vi "2013_01_04 Durability8 Main.vi"() -> ()   [LabVIEW 2011]
uses:
  MotorTypeDef.ctl
  <vilib>/DAQmx/write.llb/DAQmx Write (Counter Time 1Chan 1Samp).vi
  <vilib>/DAQmx/read.llb/DAQmx Read (Analog 1D Wfm NChan NSamp).vi
  <vilib>/Utility/TradDaqScaling.llb/Convert Thermistor Reading (waveform).vi
  <vilib>/DAQmx/miscellaneous.llb/DAQmx Fill In Error Info.vi
  <vilib>/measure/madcrms.llb/Averaged DC-RMS for N Chan.vi
  <vilib>/measure/NI_MAPro.lvlib
panel:
  out "error out":errorcluster
  in  "File Path":path=path "Durability/fine.lvm"
  out "Voltages":waveform(dbl)[](graph)
  out "Currents":waveform(dbl)[](graph)
  in  "Motor 8":T1 {"Elapsed Time" format="%<%H:%M:%S>t"; "Efficiency" format="%#_3g%%"; "Supply Voltage (V)" format="%#_3f"; "Power Output (W)" format="%#_3g"; "Power Usage (W)" format="%#_3g"; "Torque (mNm)" format="%#_3g"; "RPM" scale=0.0..40000.0 scale format="%#.6p"}
  in  "Motor 7":T1 {"Elapsed Time" format="%<%H:%M:%S>t"; "Efficiency" format="%#_3g%%"; "Supply Voltage (V)" format="%#_3f"; "Power Output (W)" format="%#_3g"; "Power Usage (W)" format="%#_3g"; "Torque (mNm)" format="%#_3g"; "RPM" scale=0.0..40000.0 scale format="%#.6p"}
  in  "Motor 6":T1 {"Elapsed Time" format="%<%H:%M:%S>t"; "Efficiency" format="%#_3g%%"; "Supply Voltage (V)" format="%#_3f"; "Power Output (W)" format="%#_3g"; "Power Usage (W)" format="%#_3g"; "Torque (mNm)" format="%#_3g"; "RPM" scale=0.0..40000.0 scale format="%#.6p"}
  in  "Motor 5":T1 {"Elapsed Time" format="%<%H:%M:%S>t"; "Efficiency" format="%#_3g%%"; "Supply Voltage (V)" format="%#_3f"; "Power Output (W)" format="%#_3g"; "Power Usage (W)" format="%#_3g"; "Torque (mNm)" format="%#_3g"; "RPM" scale=0.0..40000.0 scale format="%#.6p"}
  in  "Motor 4":T1 {"Elapsed Time" format="%<%H:%M:%S>t"; "Efficiency" format="%#_3g%%"; "Supply Voltage (V)" format="%#_3f"; "Power Output (W)" format="%#_3g"; "Power Usage (W)" format="%#_3g"; "Torque (mNm)" format="%#_3g"; "RPM" scale=0.0..40000.0 scale format="%#.6p"}
  in  "Motor 3":T1 {"Elapsed Time" format="%<%H:%M:%S>t"; "Efficiency" format="%#_3g%%"; "Supply Voltage (V)" format="%#_3f"; "Power Output (W)" format="%#_3g"; "Power Usage (W)" format="%#_3g"; "Torque (mNm)" format="%#_3g"; "RPM" scale=0.0..40000.0 scale format="%#.6p"}
  in  "Motor 2":T1 {"Elapsed Time" format="%<%H:%M:%S>t"; "Efficiency" format="%#_3g%%"; "Supply Voltage (V)" format="%#_3f"; "Power Output (W)" format="%#_3g"; "Power Usage (W)" format="%#_3g"; "Torque (mNm)" format="%#_3g"; "RPM" scale=0.0..40000.0 scale format="%#.6p"}
  in  "Motor 1":T1 {"Elapsed Time" format="%<%H:%M:%S>t"; "Efficiency" format="%#_3g%%"; "Supply Voltage (V)" format="%#_3f"; "Power Output (W)" format="%#_3g"; "Power Usage (W)" format="%#_3g"; "Torque (mNm)" format="%#_3g"; "RPM" scale=0.0..40000.0 scale format="%#.6p"}
  out "Motor Temp":dbl(slide) scale=90.0..110.0
  out "Tank Temp":dbl(slide) scale=90.0..110.0
  out "RMS Voltages":waveform(dbl)[](graph)
  out "RMS Currents":waveform(dbl)[](graph)
  in  "Temp Probe\nOn Motor":dbl=1.0
  out "loop time (ms)":u32
  in  "stop":bool
  in  "Unlock PWM":bool=TRUE
  in  "PWM 2":dbl(slide)=100.0 min=0.0 max=100.0 step=5.0 scale=0.0..100.0
  in  "PWM 1":dbl(slide) min=0.0 max=100.0 step=5.0 scale=0.0..100.0
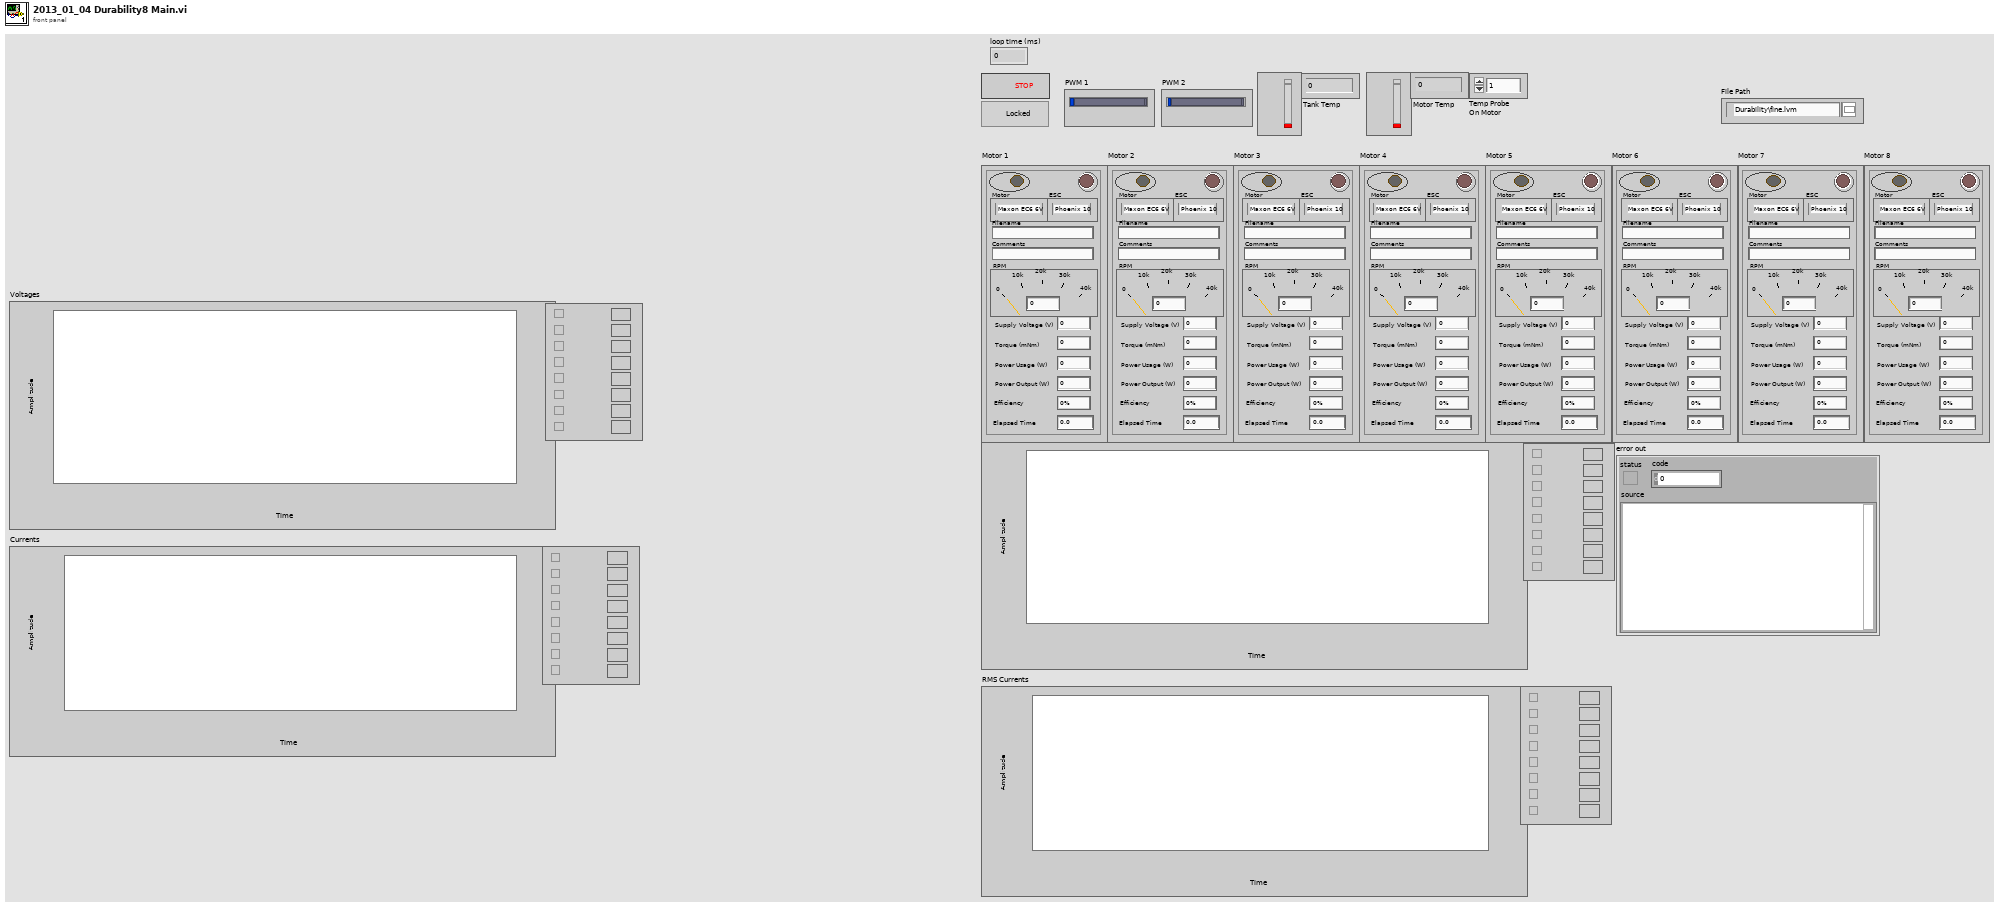
[diagram p1: front panel]
types:
  T1 = typedef "MotorTypeDef.ctl" = cluster{"Enabled":bool, "Fail":bool, "RPM":dbl, "Motor":enum16{"Maxon EC6 6V", "Maxon EC4 6V", "FH 0620 6V", "FH 0620 12V"}, "ESC":enum16{"Phoenix 10", "Maxon", "FH 1801"}, "Torque (mNm)":dbl, "Power Usage (W)":dbl, "Power Output (W)":dbl, "Supply Voltage (V)":dbl, "Efficiency":dbl, "Filename":string, "Comments":string, "Elapsed Time":dbl, "Counter":dbl}
  T2 = enum8{"Enabled", "Disabled", "Disabled and Grayed Out"}
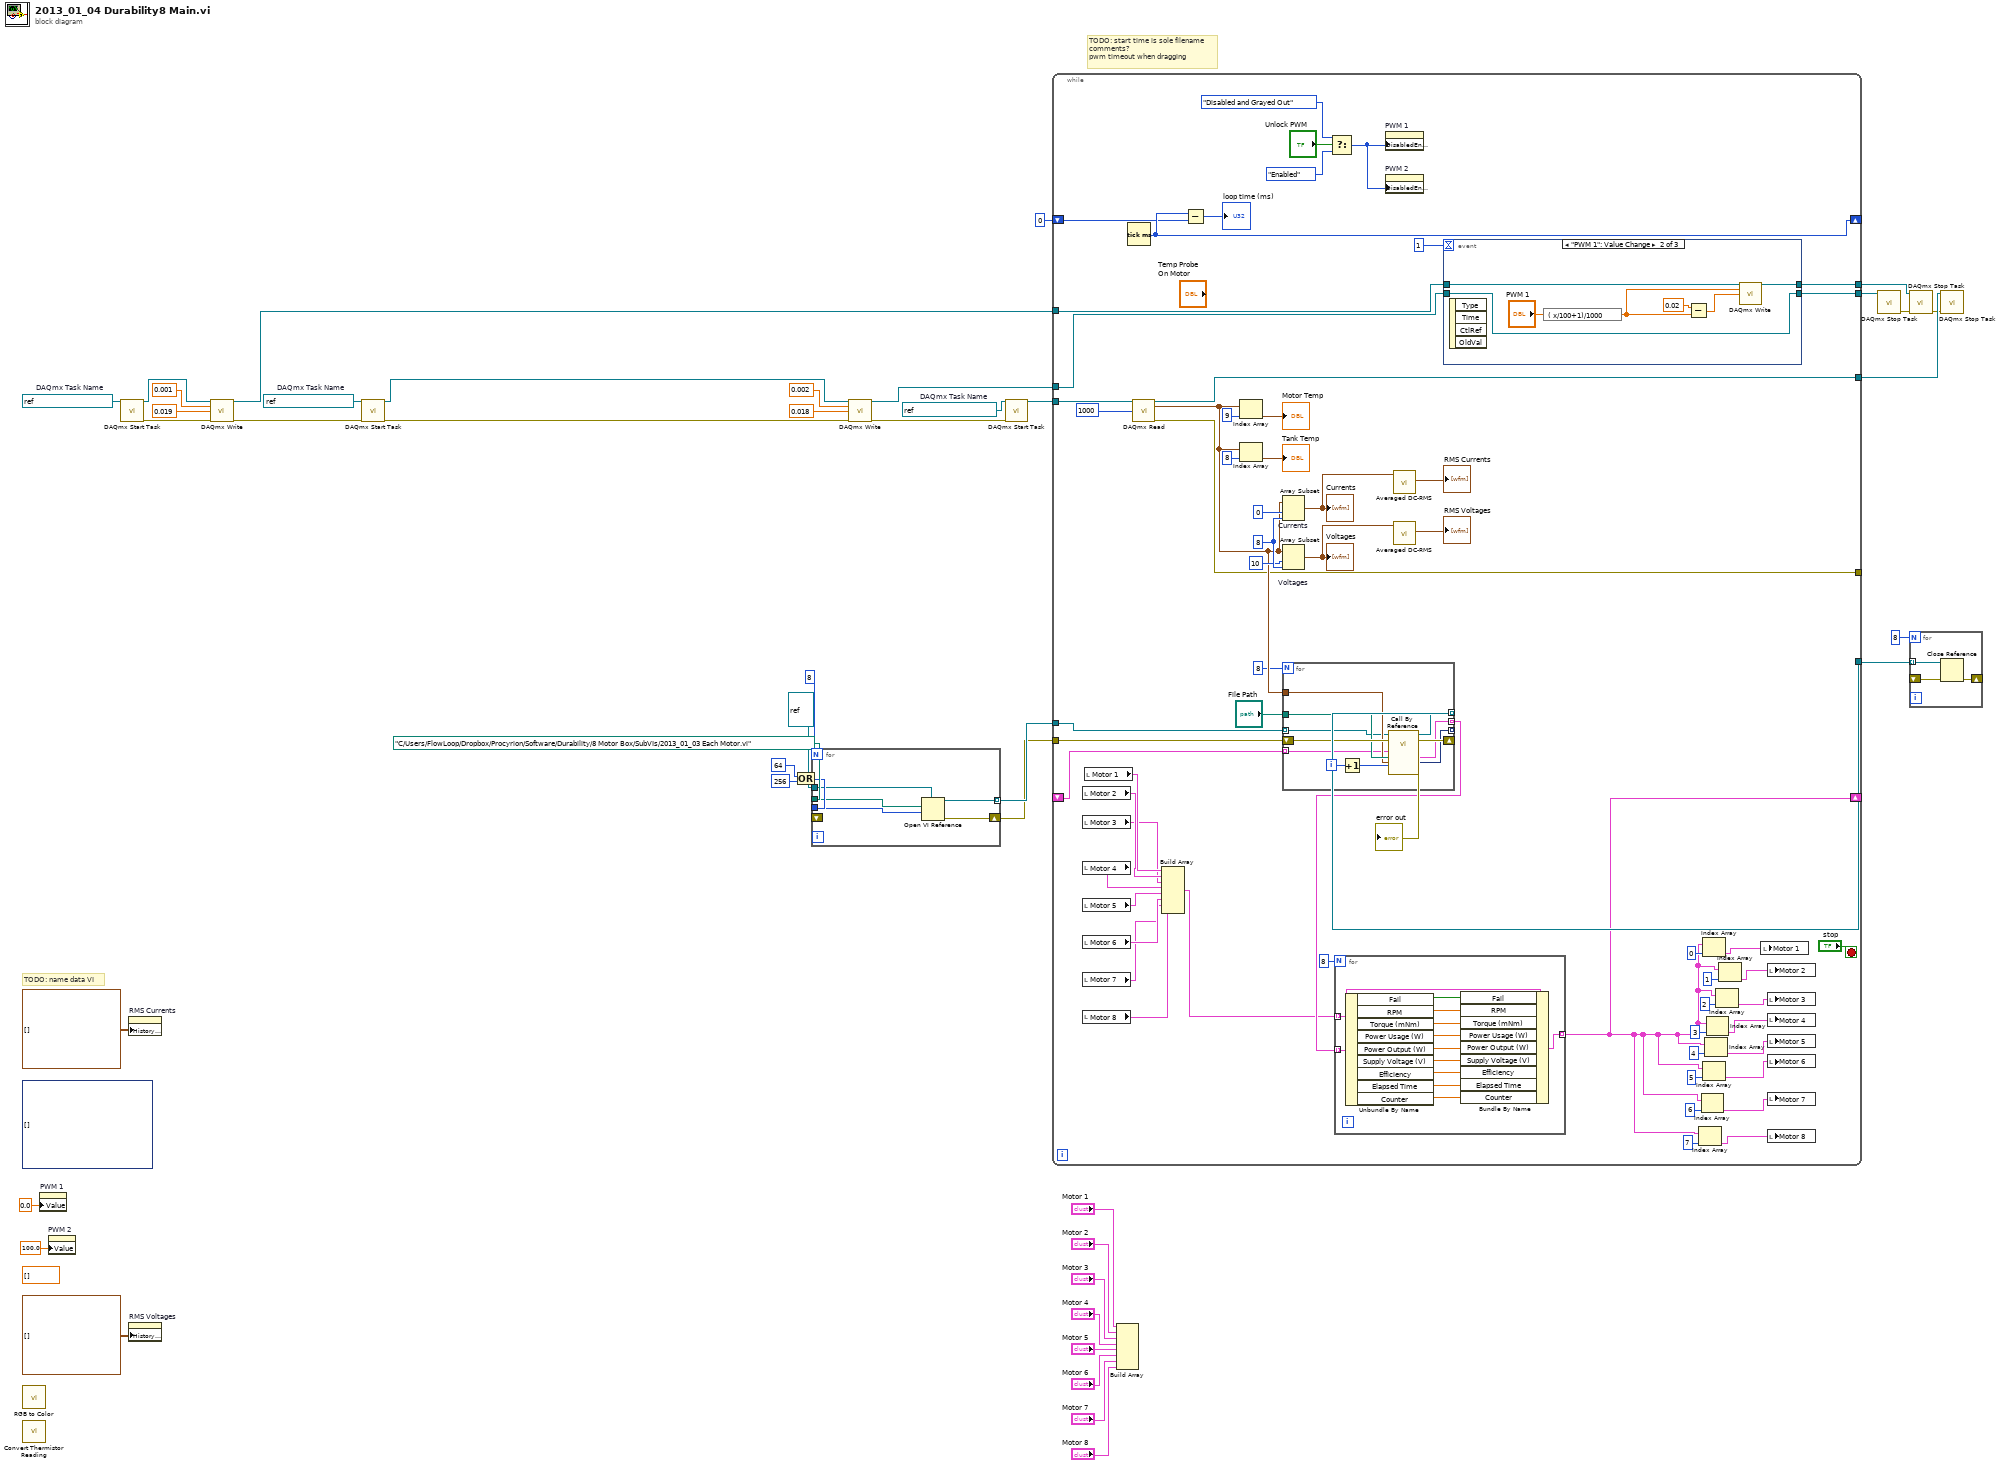
[diagram p0: block diagram]
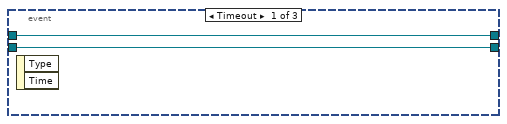
[diagram p2: hidden frame]
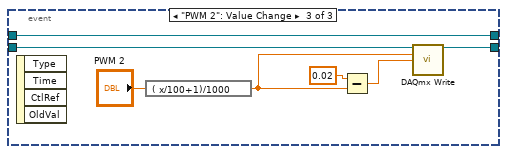
[diagram p3: hidden frame]
diagram:
  (unwired) dynamicdata[] []
  (unwired) dbl[] [] ("History Data")
  w40 = refnum<k21> "Durability8 PWM2"  # DAQmx Task Name
  w41 = refnum<k21> "Durability8 PWM1"  # DAQmx Task Name
  w44 = refnum<k21> "Durability8 Acquire"  # DAQmx Task Name
  # "TODO: start time is sole filename\ncomments?\npwm timeout when dragging"
  # "TODO: name data VI"
  n1 = call <vilib>:"RGB to Color.vi"() -> ()  [unwired: 3 in, 1 out]
  n2 = call-poly <vilib>:"Convert Thermistor Reading.vi"() -> ()  [unwired: 7 in, 1 out]
  n3 = property on="PWM 1" class="Slide (strict)"("Value"=0.0 ("PWM 1")) -> ()  [unwired: 2 in, 2 out]
  n4 = property on="PWM 2" class="Slide (strict)"("Value"=100.0 ("PWM 2")) -> ()  [unwired: 2 in, 2 out]
  n5 = call <vilib>:"DAQmx Start Task.vi"("task/channels in"=w41) -> ("task out"=w37:refnum<k21>, "error out"=w35:errorcluster)  [unwired: 13 in]
  n6 = property on="RMS Currents" class="WFChart (strict)"("History Data"=waveform(dbl)[][] []) -> ()  [unwired: 2 in, 2 out]
  n7 = property on="RMS Voltages" class="WFChart (strict)"("History Data"=waveform(dbl)[][] []) -> ()  [unwired: 2 in, 2 out]
  n8 = call-poly <vilib>:"DAQmx Write.vi"("task/channels in"=w37, "high time"=0.001 ("data"), "low time"=0.019 ("data"), "error in"=w35) -> ("task out"=w39:refnum<k21>, "error out"=w34:errorcluster)  [unwired: 9 in, 1 out]
  n9 = call <vilib>:"DAQmx Start Task.vi"("task/channels in"=w40, "error in"=w34) -> ("task out"=w36:refnum<k21>, "error out"=w33:errorcluster)  [unwired: 12 in]
  n10 = Compound Arithmetic op=OR(64 ("options"), 256 ("options")) -> (w15:i32)
  n11 = for {
    N: 8 -> [_]
    tunnel: path "C:/Users/FlowLoop/Dropbox/Procyrion/Software/Durability/8 Motor Box/SubVIs/2013_01_03 Each Motor.vi" -> [w49]
    tunnel: w15 -> [w48]
    tunnel: [w47] -> w14 mode=indexing
    tunnel: refnum<vi> refnum ("type specifier VI Refnum (for type only)") -> [w46]
    shift-right: [w45] -> w12
    shift-left: _ -> [_]
    n12 = Open VI Reference(type specifier VI Refnum (for type only)=w46, vi path=w49, options=w48) -> (vi reference=w47:refnum<vi>, error out=w45:errorcluster)  [unwired: 3 in]
  }
  n13 = call-poly <vilib>:"DAQmx Write.vi"("task/channels in"=w36, "high time"=0.002 ("data"), "low time"=0.018 ("data"), "error in"=w33) -> ("task out"=w38:refnum<k21>, "error out"=w32:errorcluster)  [unwired: 9 in, 1 out]
  n14 = call <vilib>:"DAQmx Start Task.vi"("task/channels in"=w44, "error in"=w32) -> ("task out"=w43:refnum<k21>)  [unwired: 12 in, 1 out]
  n15 = while {
    tunnel: w43 -> [w113]
    tunnel: [w112] -> w42
    tunnel: w12 -> [w82]
    shift-right: [w106] -> _
    shift-left: u32 0 ("millisecond timer value") -> [w105]
    tunnel: w39 -> [w92]
    tunnel: w38 -> [w91]
    tunnel: [w90] -> w31
    tunnel: [w89] -> w22
    tunnel: w14 -> [w83]
    tunnel: [w80] -> _
    tunnel: [w79] -> w9
    shift-right: [w51] -> _
    shift-left: _ -> [w50]
    stop <- "stop" stop-if-true
    w101 = 8 ("length")
    n16 = local read "Motor 2"() -> (w59:T1)
    n17 = local read "Motor 3"() -> (w58:T1)
    n18 = local read "Motor 4"() -> (w57:T1)
    n19 = local read "Motor 5"() -> (w56:T1)
    n20 = local read "Motor 6"() -> (w55:T1)
    n21 = local read "Motor 7"() -> (w54:T1)
    n22 = local read "Motor 8"() -> (w53:T1)
    n23 = local read "Motor 1"() -> (w60:T1)
    n24 = Tick Count (ms)() -> (millisecond timer value=w106:u32)
    n25 = call-poly <vilib>:"DAQmx Read.vi"("task/channels in"=w113, "number of samples per channel"=1000) -> ("task out"=w112:refnum<k21>, "data"=w94:waveform(dbl)[], "error out"=w80:errorcluster)  [unwired: 11 in]
    n26 = Build Array(w60, w59, w58, w57, w56, w55, w54, w53) -> (w52:T1[])
    n27 = Subtract(x=w106, y=w105) -> (x-y=→"loop time (ms)":u32)
    n28 = Index Array(array=w94, index=9) -> (element=→"Motor Temp":waveform(dbl))
    n29 = Index Array(array=w94, index=8) -> (element=→"Tank Temp":waveform(dbl))
    n30 = Array Subset "Currents"(array=w94, index=0, length=w101) -> (w87:waveform(dbl)[])
    "Currents" <- w87
    n31 = Array Subset "Voltages"(array=w94, index=10 ("length"), length=w101) -> (w86:waveform(dbl)[])
    "Voltages" <- w86
    n32 = for {
      N: 8 -> [_]
      tunnel: w94 -> [w148]
      tunnel: "File Path" -> [w149]
      tunnel: w83 -> [w145] mode=indexing
      shift-right: [w152] -> w81
      shift-left: w82 -> [w151]
      tunnel: [w146] -> _ mode=indexing
      tunnel: [w144] -> w79 mode=indexing
      tunnel: [w143] -> w77 mode=indexing
      tunnel: w50 -> [w142] mode=indexing
      i -> [w150]
      n33 = Increment(x=w150) -> (x+1=w147:i32)
      n34 = call-by-ref "?"(reference=w145, error in=w151, "Motor #"=w147, "data"=w148, "File Path"=w149, "Motor Typedef"=w142) -> (reference out=w144:refnum<vi>, error out=w152:errorcluster, "Waveform Graph"=w146:dynamicdata, "Motor Typedef Out"=w143:T1)  [unwired: 3 in, 1 out]
    }
    "error out" <- w81
    n35 = Select(t=T2."Disabled and Grayed Out" ("Disabled"), s="Unlock PWM", f=T2."Enabled" ("Disabled")) -> (s? t:f=w110:T2)
    n36 = for {
      N: 8 -> [_]
      tunnel: w52 -> [w116] mode=indexing
      tunnel: [w115] -> w51 mode=indexing
      tunnel: w77 -> [w114] mode=indexing
      n37 = Unbundle By Name(w114) -> ("Fail"=w125:bool, "RPM"=w124:dbl, "Torque (mNm)"=w123:dbl, "Power Usage (W)"=w122:dbl, "Power Output (W)"=w121:dbl, "Supply Voltage (V)"=w120:dbl, "Efficiency"=w119:dbl, "Elapsed Time"=w118:dbl, "Counter"=w117:dbl)
      n38 = Bundle By Name(cluster=w116, "Fail"=w125, "RPM"=w124, "Torque (mNm)"=w123, "Power Usage (W)"=w122, "Power Output (W)"=w121, "Supply Voltage (V)"=w120, "Efficiency"=w119, "Elapsed Time"=w118, "Counter"=w117) -> (w115:T1)
    }
    n39 = property on="PWM 1" class="Slide (strict)"("DisabledEnum"=w110) -> ()  [unwired: 2 in, 2 out]
    n40 = property on="PWM 2" class="Slide (strict)"("DisabledEnum"=w110) -> ()  [unwired: 2 in, 2 out]
    n41 = call-poly <vilib>:"Averaged DC-RMS.vi"("signals in"=w87) -> ("RMS value waveforms"=→"RMS Currents":waveform(dbl)[])  [unwired: 6 in, 4 out]
    n42 = call-poly <vilib>:"Averaged DC-RMS.vi"("signals in"=w86) -> ("RMS value waveforms"=→"RMS Voltages":waveform(dbl)[])  [unwired: 6 in, 4 out]
    n43 = event shown="[1] \"PWM 1\": Value Change" {
      selector: _ -> [_ _ _]
      dyn-events: _ -> [_ _ _]
      timeout: 1 -> [_ _ _]
      tunnel: w92 -> [w127 w130 w136]
      tunnel: w91 -> [w126 w128 w135]
      tunnel: [w127 w129 w136] -> w90
      tunnel: [w126 w128 w137] -> w89
      event Timeout {
        n44 = event-data() -> ()  [unwired: 1 in, 2 out]
      }
      event "PWM 1": Value Change {
        n45 = event-data() -> ()  [unwired: 1 in, 4 out]
        n46 = expression code="( x/100+1)/1000"("PWM 1") -> (w131:dbl)
        n47 = Subtract(x=0.02 ("y"), y=w131) -> (x-y=w132:dbl)
        n48 = call-poly <vilib>:"DAQmx Write.vi"("task/channels in"=w130, "high time"=w131, "low time"=w132) -> ("task out"=w129:refnum<k21>)  [unwired: 10 in, 2 out]
      }
      event "PWM 2": Value Change {
        n49 = event-data() -> ()  [unwired: 1 in, 4 out]
        n50 = expression code="( x/100+1)/1000"("PWM 2") -> (w141:dbl)
        n51 = Subtract(x=0.02, y=w141) -> (x-y=w139:dbl)
        n52 = call-poly <vilib>:"DAQmx Write.vi"("task/channels in"=w135, "high time"=w141, "low time"=w139) -> ("task out"=w137:refnum<k21>)  [unwired: 10 in, 2 out]
      }
    }
    n53 = Index Array(array=w51, index=7) -> (element=w67:T1)
    n54 = Index Array(array=w51, index=6) -> (element=w66:T1)
    n55 = Index Array(array=w51, index=0) -> (element=w76:T1)
    n56 = Index Array(array=w51, index=5) -> (element=w65:T1)
    n57 = Index Array(array=w51, index=4) -> (element=w64:T1)
    n58 = Index Array(array=w51, index=3) -> (element=w63:T1)
    n59 = Index Array(array=w51, index=2) -> (element=w62:T1)
    n60 = Index Array(array=w51, index=1) -> (element=w61:T1)
    n61 = local write "Motor 1"(w76) -> ()
    n62 = local write "Motor 2"(w61) -> ()
    n63 = local write "Motor 3"(w62) -> ()
    n64 = local write "Motor 4"(w63) -> ()
    n65 = local write "Motor 5"(w64) -> ()
    n66 = local write "Motor 6"(w65) -> ()
    n67 = local write "Motor 7"(w66) -> ()
    n68 = local write "Motor 8"(w67) -> ()
  }
  n69 = Build Array("Motor 1", "Motor 2", "Motor 3", "Motor 4", "Motor 5", "Motor 6", "Motor 7", "Motor 8") -> ()  [unwired: 1 out]
  n70 = call <vilib>:"DAQmx Stop Task.vi"("task/channels in"=w22) -> ("error out"=w30:errorcluster)  [unwired: 13 in, 1 out]
  n71 = call <vilib>:"DAQmx Stop Task.vi"("task/channels in"=w31, "error in"=w30) -> ("error out"=w29:errorcluster)  [unwired: 12 in, 1 out]
  n72 = for {
    N: 8 -> [_]
    shift-right: [w155] -> _
    shift-left: _ -> [w153]
    tunnel: w9 -> [w154] mode=indexing
    n73 = Close Reference(reference=w154, error in (no error)=w153) -> (error out=w155:errorcluster)
  }
  n74 = call <vilib>:"DAQmx Stop Task.vi"("task/channels in"=w42, "error in"=w29) -> ()  [unwired: 12 in, 2 out]
